vi "VSM9T_Splitt_Cluster.vi"(0 "VSM-9T-Cluster":T3 {"Rate (T/min)" format="%6_5f"; "Leads (T)" format="%6_5f"}) -> (1 "VSM-9T-Status-Cluster":T1 {"Leads (T)" format="%6_5f"}, 2 "VSM-9T-Control-Cluster":T2 {"Rate (T/min)" format="%6_5f"})   [LabVIEW 2019]
uses:
  VSM/VSM9T-Cluster.ctl
  VSM/VSM9T-Control-Cluster.ctl
  VSM/VSM9T-Status-Cluster.ctl
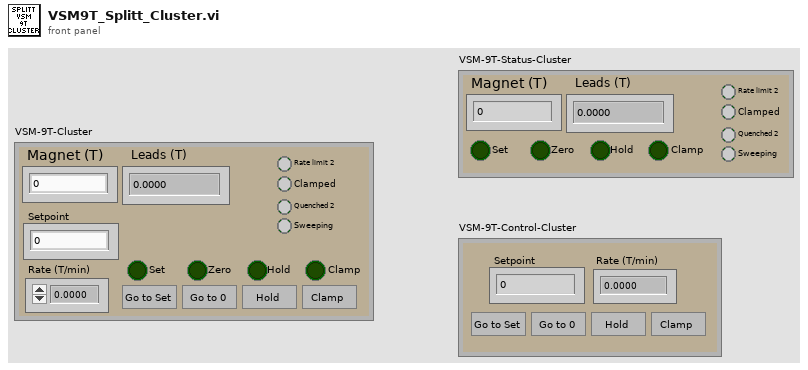
[diagram p1: front panel]
types:
  T1 = typedef "VSM9T-Status-Cluster.ctl" = cluster{"Clamped ":bool, "Quenched 2":bool, "Rate limit 2":bool, "Magnet (T)":dbl, "Leads (T)":dbl, "Sweeping":bool, "Set":bool, "Zero":bool, "Hold":bool, "Clamp":bool}
  T2 = typedef "VSM9T-Control-Cluster.ctl" = cluster{"Go to set":bool, "Go to Zero":bool, "Clamp":bool, "Go to Hold":bool, "Rate (T/min)":dbl, "Setpoint":dbl}
  T3 = typedef "VSM9T-Cluster.ctl" = cluster{"Go to set":bool, "Go to Zero":bool, "Clamp":bool, "Go to Hold":bool, "Clamped ":bool, "Quenched 2":bool, "Rate limit 2":bool, "Magnet (T)":dbl, "Leads (T)":dbl, "Rate (T/min)":dbl, "Sweeping":bool, "Setpoint":dbl, "Set":bool, "Zero":bool, "Hold":bool, "Clamp":bool}
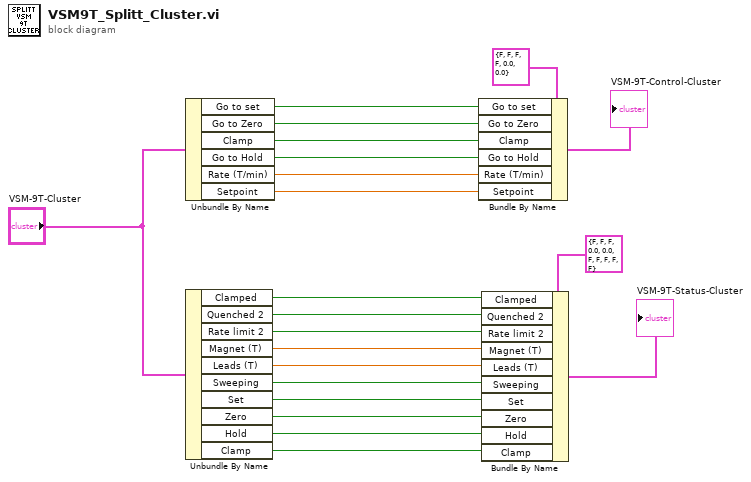
[diagram p0: block diagram]
diagram:
  n1 = Unbundle By Name("VSM-9T-Cluster") -> ("Go to set"=w17:bool, "Go to Zero"=w16:bool, "Clamp"=w15:bool, "Go to Hold"=w14:bool, "Rate (T/min)"=w13:dbl, "Setpoint"=w12:dbl)
  n2 = Unbundle By Name("VSM-9T-Cluster") -> ("Clamped"=w10:bool, "Quenched 2"=w9:bool, "Rate limit 2"=w8:bool, "Magnet (T)"=w7:dbl, "Leads (T)"=w6:dbl, "Sweeping"=w5:bool, "Set"=w4:bool, "Zero"=w3:bool, "Hold"=w2:bool, "Clamp"=w1:bool)
  n3 = Bundle By Name(cluster=T2 {"Go to set"=FALSE, "Go to Zero"=FALSE, "Clamp"=FALSE, "Go to Hold"=FALSE, "Rate (T/min)"=0.0, "Setpoint"=0.0} ("VSM-9T-Control-Cluster"), "Go to set"=w17, "Go to Zero"=w16, "Clamp"=w15, "Go to Hold"=w14, "Rate (T/min)"=w13, "Setpoint"=w12) -> (→"VSM-9T-Control-Cluster":T2)
  n4 = Bundle By Name(cluster=T1 {"Clamped "=FALSE, "Quenched 2"=FALSE, "Rate limit 2"=FALSE, "Magnet (T)"=0.0, "Leads (T)"=0.0, "Sweeping"=FALSE, "Set"=FALSE, "Zero"=FALSE, "Hold"=FALSE, "Clamp"=FALSE} ("VSM-9T-Status-Cluster"), "Clamped"=w10, "Quenched 2"=w9, "Rate limit 2"=w8, "Magnet (T)"=w7, "Leads (T)"=w6, "Sweeping"=w5, "Set"=w4, "Zero"=w3, "Hold"=w2, "Clamp"=w1) -> (→"VSM-9T-Status-Cluster":T1)
